vi "TestIddLowPower.vi"(5 "Deep Sleep Time":u32, 6 "channel name":string="0", 7 "Active Dut":T1, 8 "Error In":errorcluster, 9 "Resp Timeout (ms)":i32=1000, 10 "FPGA Reference":refnum<k20>, 11 "SMU Handle":refnum<k15>) -> (0 "error out":errorcluster, 2 "Idd Average":dbl)   [LabVIEW 2018]
uses:
  Resources_Test/UART/ControlTestSlot.ctl
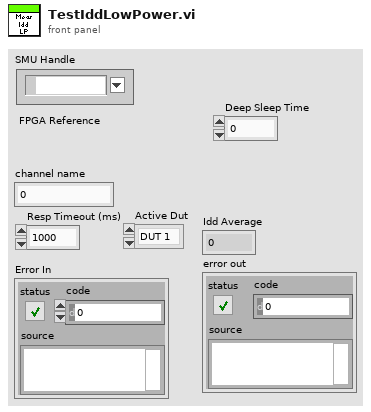
[diagram p1: front panel]
types:
  T1 = typedef "ControlTestSlot.ctl" = enum16{"DUT 1", "DUT 2"}
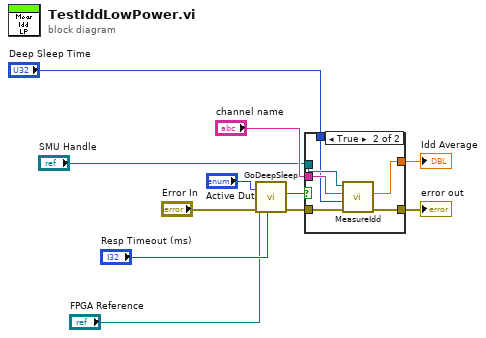
[diagram p0: block diagram]
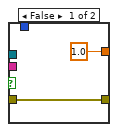
[diagram p2: hidden frame]
diagram:
  n1 = call "GoDeepSleep.vi"("Resp Timeout (ms)"="Resp Timeout (ms)", "Enum"="Active Dut", "Error In"="Error In", "FPGA Reference"="FPGA Reference") -> ("Error Out"=w9:errorcluster, "Deep Sleep OK"=w10:bool)  [unwired: 5 in, 1 out]
  n2 = case shown="True" w10 {
    tunnel: [1.0 ("Idd Average") w19] -> w5
    tunnel: [w13 w18] -> w4
    tunnel: w9 -> [w13 w17]
    tunnel: "channel name" -> [_ w16]
    tunnel: "SMU Handle" -> [_ w15]
    tunnel: "Deep Sleep Time" -> [_ w14]
    frame False {
    }
    frame True {
      n3 = call "MeasureIdd.vi"("error in (no error)"=w17, "Deep Sleep Time"=w14, "channel name"=w16, "instrument handle"=w15) -> ("error out"=w18:errorcluster, "Idd Average"=w19:dbl)  [unwired: 5 in, 1 out]
    }
  }
  "Idd Average" <- w5
  "error out" <- w4
